vi "ErrorHandlerGFV.vi"(7 "?":T1, 8 "error in (no error)":errorcluster, 9 "Display Queue":refnum<queue>, 10 "Consumer Queue":refnum<queue>, 11 "user event out":refnum<user-event>) -> (0 "error out":errorcluster)   [LabVIEW 2013]
doc: "Use this template to build a VI to use as a subVI."
uses:
  TypeDef/DisplayQueue.ctl
  TypeDef/DisplayEnum.ctl
  TypeDef/ConsumerQueue.ctl
  TypeDef/ConsumerEnum.ctl
  TypeDef/ErrorHandleEnum.ctl
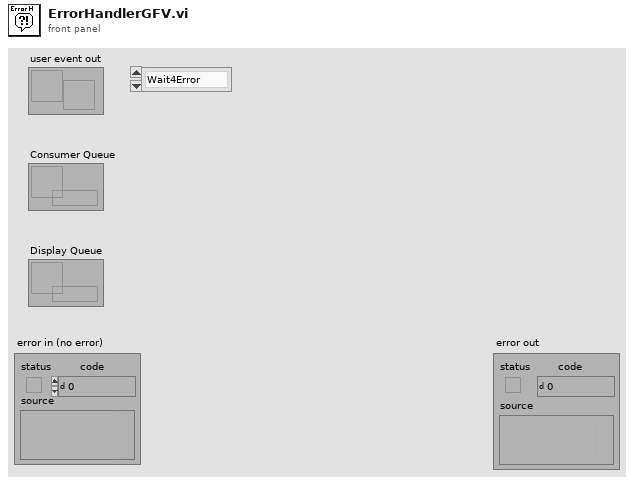
[diagram p1: front panel]
types:
  T1 = typedef "ErrorHandleEnum.ctl" = enum16{"Wait4Error", "Init"}
  T2 = typedef "DisplayEnum.ctl" = enum16{"Stop Display", "Update Display", "Update Multiple Files Display", "Center Image", "Update Configuration Display", "Init Display"}
  T3 = typedef "ConsumerEnum.ctl" = enum16{"Init Error Handler", "Init Configuration DB", "Init Droplet DB", "Stop", "Detect Freeze", "Stop Freeze Detection", "Open DropletDB", "DisplayImageNumber", "Save DropletDB", "UpdateFileIndices", "UpdateInlcudeDroplet", "Insert Configuration Data", "Detect Droplets"}
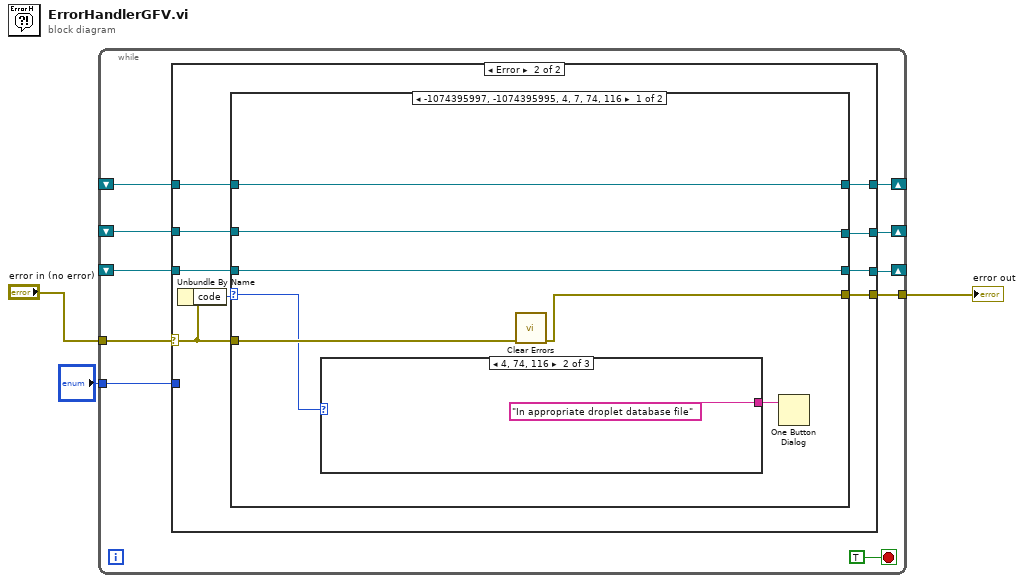
[diagram p0: block diagram]
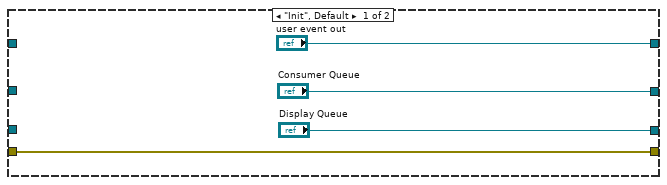
[diagram p3: hidden frame]
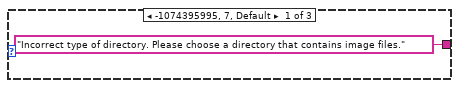
[diagram p4: hidden frame]
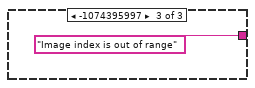
[diagram p5: hidden frame]
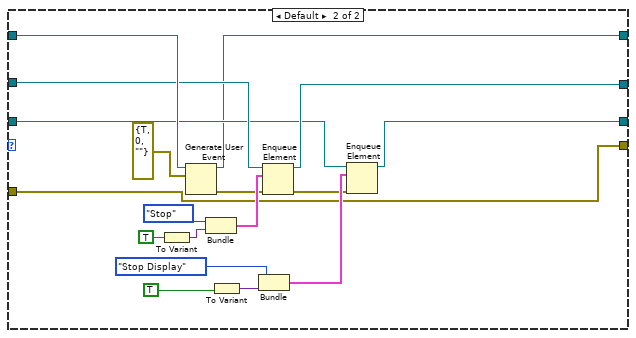
[diagram p6: hidden frame]
diagram:
  n1 = while {
    tunnel: "?" -> [w12]
    tunnel: "error in (no error)" -> [w8]
    shift-right: [w11] -> _
    shift-left: _ -> [w7]
    shift-right: [w10] -> _
    shift-left: _ -> [w6]
    shift-right: [w9] -> _
    shift-left: _ -> [w5]
    tunnel: [w4] -> w1
    stop <- TRUE stop-if-true
    n2 = case shown="Error" w8 {
      selector: w8 -> [w17 w34]
      tunnel: w12 -> [w22 _]
      tunnel: [w21 w31] -> w11
      tunnel: [w20 w37] -> w10
      tunnel: [w19 w35] -> w9
      tunnel: w7 -> [w16 w39]
      tunnel: w6 -> [w15 w38]
      tunnel: w5 -> [w14 w36]
      tunnel: [w18 w32] -> w4
      frame No Error {
        n3 = case shown="\"Wait4Error\"" w22 {
          tunnel: ["user event out" w30] -> w21
          tunnel: ["Consumer Queue" w29] -> w20
          tunnel: ["Display Queue" w28] -> w19
          tunnel: [w23 w27] -> w18
          tunnel: w17 -> [w23 w27]
          tunnel: w16 -> [_ w30]
          tunnel: w15 -> [_ w29]
          tunnel: w14 -> [_ w28]
          frame "Init", Default {
          }
          frame "Wait4Error" {
          }
        }
      }
      frame Error {
        n4 = Unbundle By Name(w34) -> ("code"=w33:i32)
        n5 = case shown="-1074395997, -1074395995, 4, 7, 74, 116" w33 {
          selector: w33 -> [w40 _]
          tunnel: w39 -> [w46 w67]
          tunnel: w38 -> [w45 w61]
          tunnel: [w45 w60] -> w37
          tunnel: w36 -> [w44 w53]
          tunnel: [w44 w52] -> w35
          tunnel: w34 -> [w43 w51]
          tunnel: [w42 w51] -> w32
          tunnel: [w46 w50] -> w31
          frame -1074395997, -1074395995, 4, 7, 74, 116 {
            n6 = case shown="4, 74, 116" w40 {
              tunnel: ["Incorrect type of directory. Please choose a directory that contains image files." ("message") "In appropriate droplet database file" ("message") "Image index is out of range" ("message")] -> w41
              frame -1074395995, 7, Default {
              }
              frame 4, 74, 116 {
              }
              frame -1074395997 {
              }
            }
            n7 = call <vilib>:"Clear Errors.vi"("error in (no error)"=w43) -> ("error out"=w42:errorcluster)  [unwired: 6 in]
            n8 = One Button Dialog(message=w41) -> ()  [unwired: 1 in, 1 out]
          }
          frame Default {
            n9 = To Variant(anything=TRUE) -> (Variant=w64:variant)
            n10 = Generate User Event(user event=w67, event data cluster=errorcluster {"status"=TRUE, "code"=0, "source"=""} ("event data")) -> (user event out=w50:refnum<user-event>, error out=w59:errorcluster)  [unwired: 2 in]
            n11 = Bundle(ConsumerEnum."Stop", "Variant"=w64) -> (w63:cluster{T3, "Variant":variant})  [unwired: 1 in]
            n12 = To Variant(anything=TRUE) -> (Variant=w58:variant)
            n13 = Bundle("Enum"=DisplayEnum."Stop Display", "Variant"=w58) -> (w56:cluster{"Enum":T2, "Variant":variant})  [unwired: 1 in]
            n14 = Enqueue Element(queue=w61, element=w63, error in (no error)=w59) -> (queue out=w60:refnum<queue>, error out=w54:errorcluster)  [unwired: 1 in, 1 out]
            n15 = Enqueue Element(queue=w53, element=w56, error in (no error)=w54) -> (queue out=w52:refnum<queue>)  [unwired: 1 in, 2 out]
          }
        }
      }
    }
  }
  "error out" <- w1
